vi "Process.vi"(8 "error in":errorcluster, 11 "Instrument":refnum<class "Instrument.lvclass">) -> (0 "error out":errorcluster, 3 "Instrument out":refnum<class "Instrument.lvclass">)   [LabVIEW 2019, in "Instrument.lvclass"]
doc: "---------------------------------------------------------------\nJKI State Machine Objects™\nhttp://jki.net/state-machine-objects/\nCopyright (C) 2005-2015, JKI <info@jki.net>\nALL RIGHTS RESERVED"
uses:
  Instrument.lvclass
  <vilib>/JKI/JKI SMO/SMO/SMO.lvclass
  <userlib>/LevyLab/RemoteControl/RemoteControl.lvclass
  <userlib>/LevyLab/RemoteControl/Typedefs/Message--Cluster.ctl
  <userlib>/LevyLab/RemoteControl/Typedefs/PrivateEvents--RemoteControl.Configure.ctl
  Logger.PGSQL/Logger.PGSQL.lvclass
  Logger.PGSQL/Typedefs/PrivateEvents--Logger.PGSQL.Write Variable.ctl
  C:/Program Files (x86)/National Instruments/LabVIEW 2019/vi.lib/JKI/JKI SMO/SMO/SMO.lvclass
  Logger.Error/Logger.Error.lvclass
panel:
  out "State History":string
  out "Local Command":string
  out "Name":string
  out "Remote Command":string
  # "1. Receives & processes commands from RemoteControl process\n2. Logs instrument settings to PGSQL using Logger process"
  # "INSTRUMENT"
  # "INSTRUMENT"
  # "For instructions on how to use the JKI State Machine Objects, examples and video tutorials, visit:\nhttp://jki.net/state-machine-objects/\n\nJKI State Machine Objects™\nhttp://jki.net/state-machine-objects/\nCopyright (C) 2005-2015, JKI <info@jki.net>\nALL RIGHTS RESERVED"
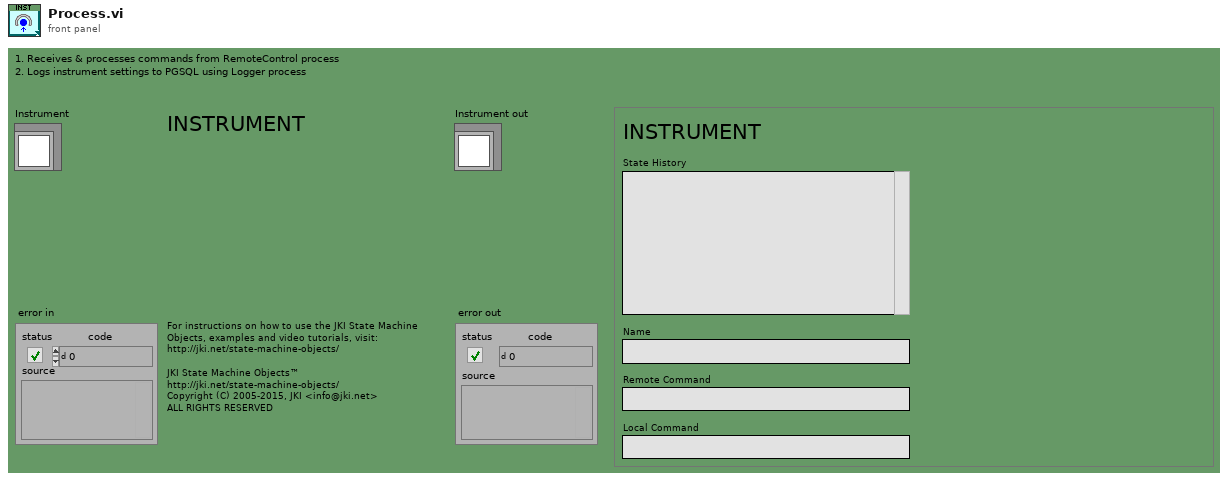
[diagram p1: front panel]
types:
  T1 = enum32{"invalid app kind", "Development System", "Run Time System", "Student Edition", "Embedded LabVIEW", "Evaluation", "Custom"}
  T2 = enum32{"Invalid", "Standard", "Closed", "Hidden", "Minimized", "Maximized"}
  T3 = typedef "RemoteControl.lvclass/Message--Cluster.ctl" = cluster{"Command":string, "Data":variant, "ID":string}
  T4 = typedef "Instrument.lvclass/Dependencies--Cluster.ctl" = cluster{"RemoteControl":refnum<class "RemoteControl.lvclass">, "Logger.Error":refnum<class "Logger.Error.lvclass">, "Logger.PGSQL":refnum<class "Logger.PGSQL.lvclass">, "Configuration":refnum<class "Configuration.lvclass">}
  T5 = typedef "RemoteControl.lvclass/PrivateEvents--RemoteControl.Configure.ctl" = cluster{"address":string, "Port":u16, "AllowedRemote":string, "Commands":string[], "timeout":i32}
  T6 = typedef "Logger.PGSQL.lvclass/PrivateEvents--Logger.PGSQL.Write Variable.ctl" = cluster{"Address":string, "Data":variant}
  T7 = cluster{"Core":cluster{"Current VI Reference":refnum<vi>, "Close Panel on Exit?":bool, "Last Error":cluster{"error":errorcluster, "previous state":string, "remaining states":string}, "Shutdown?":bool}, "SelfRef":refnum<class "Instrument.lvclass">, "Dependencies":T4, "RC Configuration":T5, "Message":T3, "getAll":variant, "Debug Mode?":bool, "PGSQL":T6}
  T8 = typedef "SMO.lvclass/SMOState --Enum.ctl" = enum16{"unknown", "Created", "Started", "Stopped"}
  T9 = cluster{"Current VI Reference":refnum<vi>, "Close Panel on Exit?":bool, "Last Error":cluster{"error":errorcluster, "previous state":string, "remaining states":string}, "Shutdown?":bool}
  T10 = typedef "SMO.lvclass/Protected Events.ctl" = cluster{"StopProcesses":refnum<user-event>, "AbortProcesses":refnum<user-event>, "Config Changed":refnum<user-event>, "Dependency":refnum<user-event>}
  T11 = typedef "Instrument.lvclass/PrivateEvents--Cluster.ctl" = cluster{"MessageToProcess":refnum<user-event>, "Log PGSQL":refnum<user-event>}
  T12 = typedef "RemoteControl.lvclass/PublicEvents--Cluster.ctl" = cluster{"SendMessageFromProcess":refnum<user-event>}
  T13 = typedef "SMO.lvclass/Public Events.ctl" = cluster{"Error":refnum<user-event>, "State":refnum<user-event>, "Reserve State":refnum<user-event>}
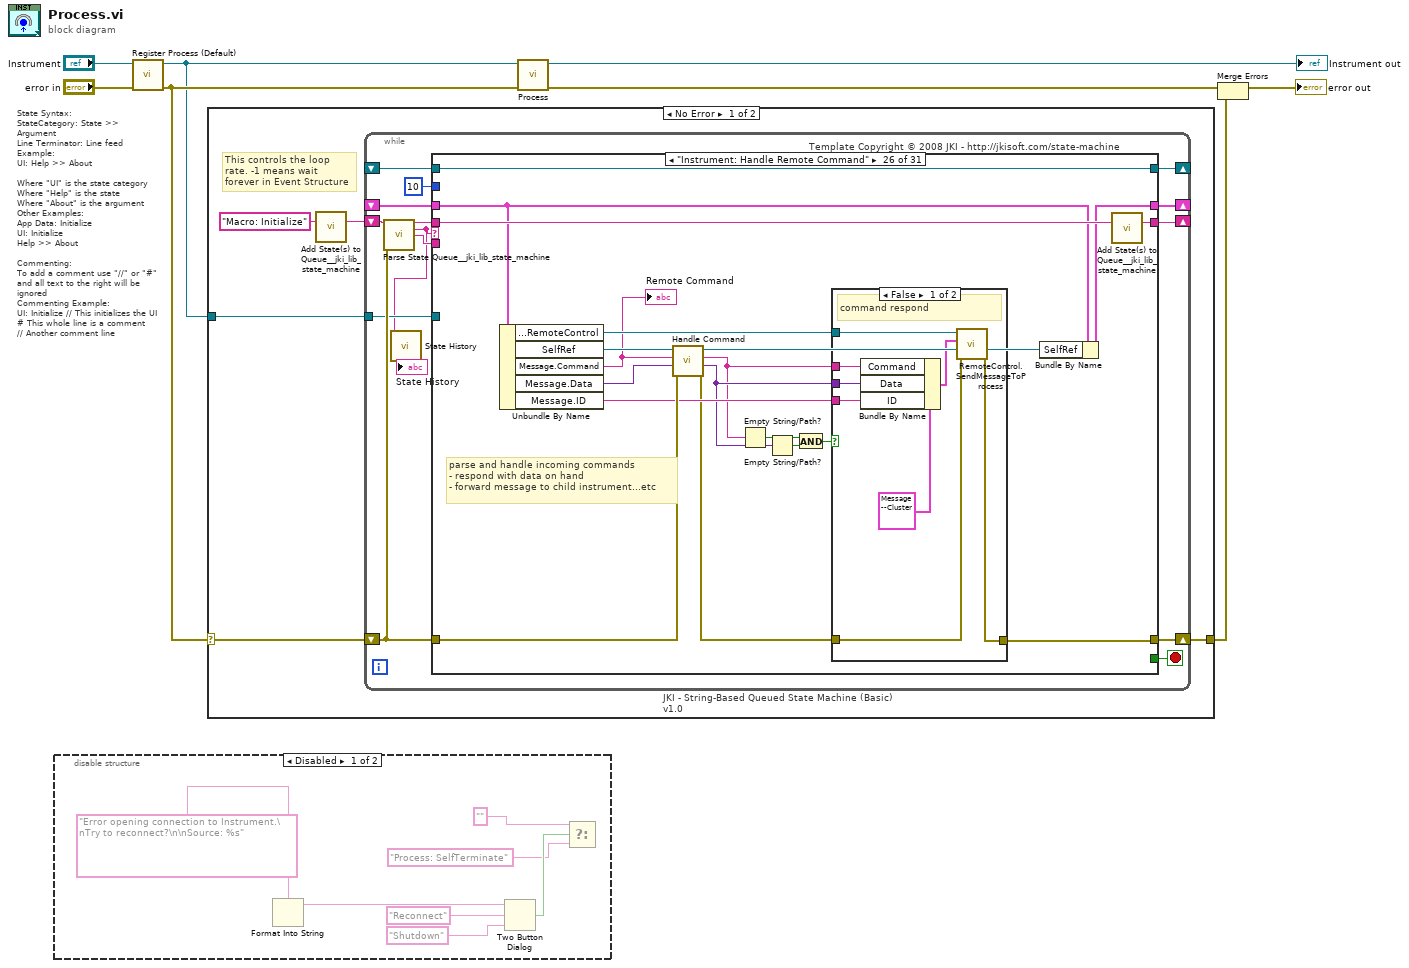
[diagram p0: block diagram]
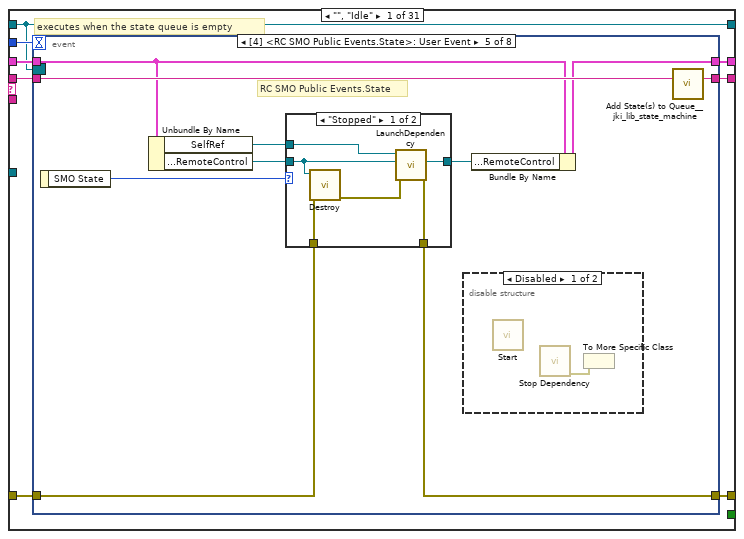
[diagram p3: hidden frame]
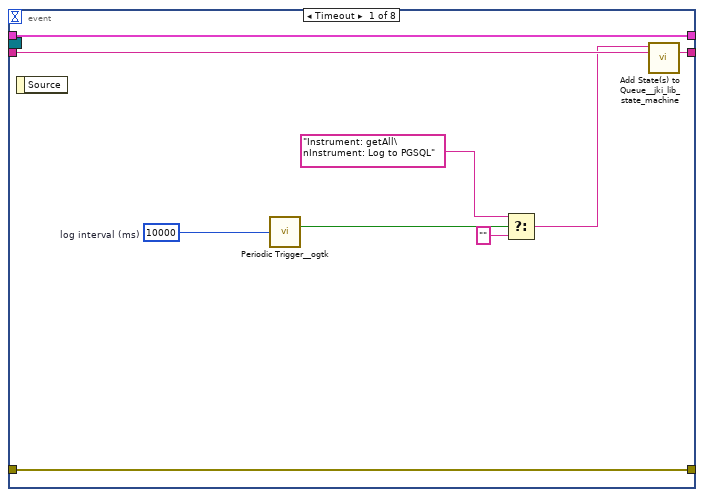
[diagram p4: hidden frame]
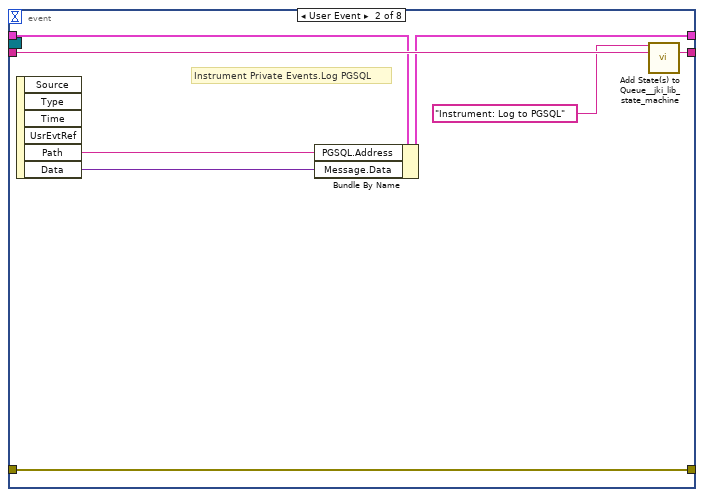
[diagram p5: hidden frame]
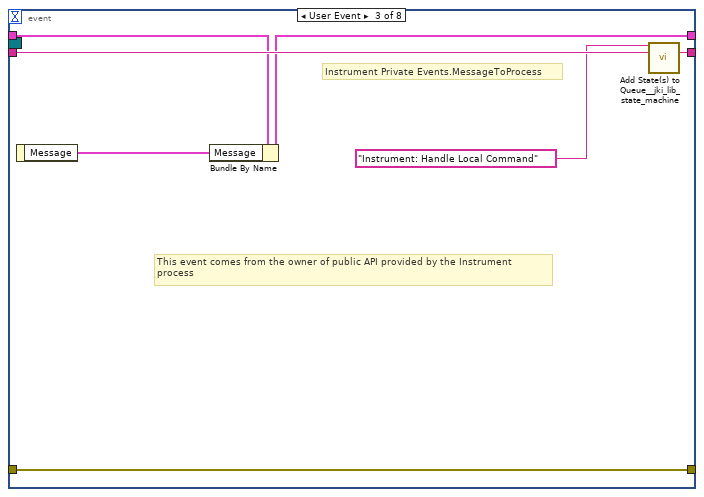
[diagram p6: hidden frame]
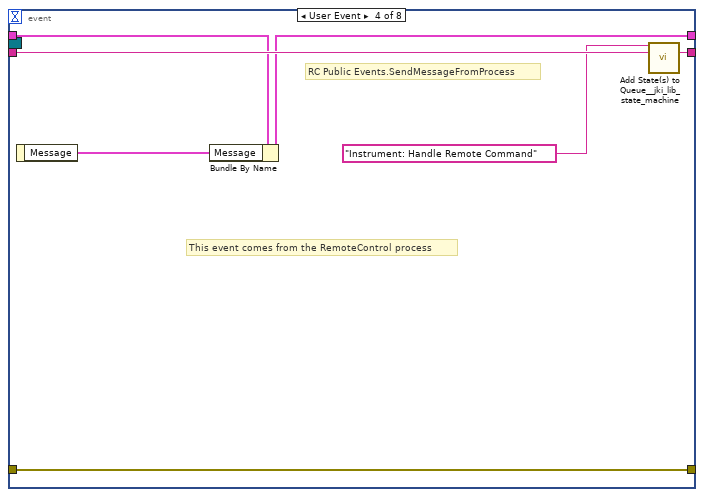
[diagram p7: hidden frame]
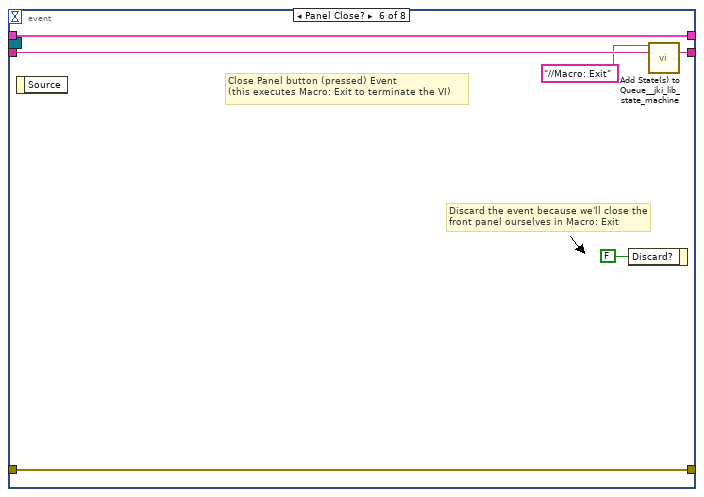
[diagram p10: hidden frame]
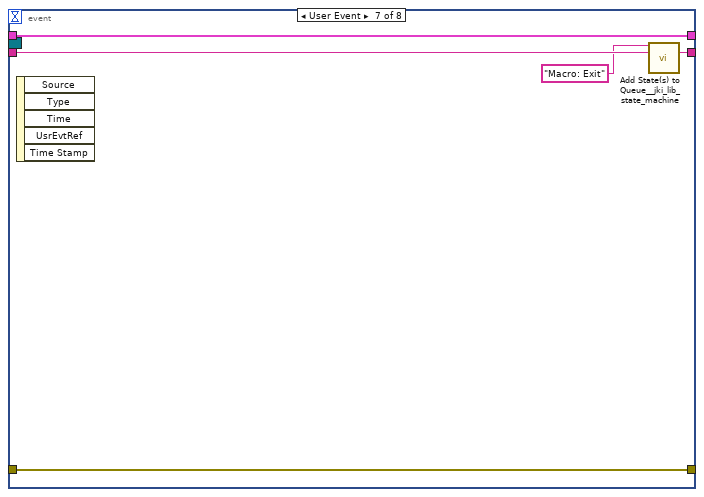
[diagram p11: hidden frame]
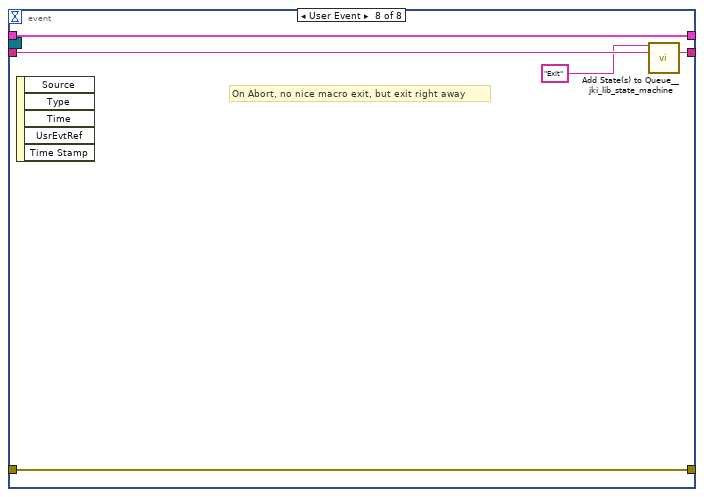
[diagram p12: hidden frame]
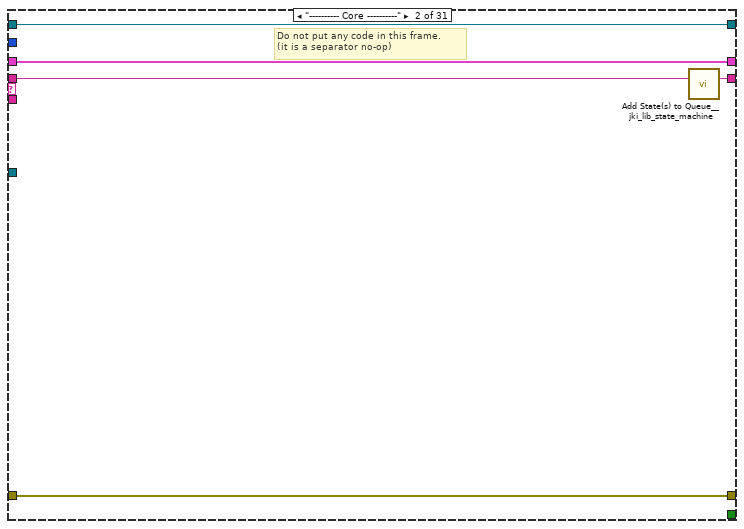
[diagram p13: hidden frame]
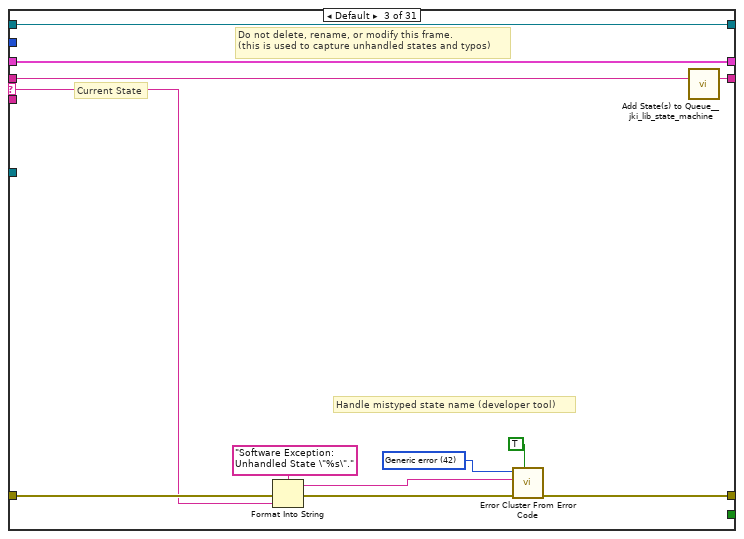
[diagram p14: hidden frame]
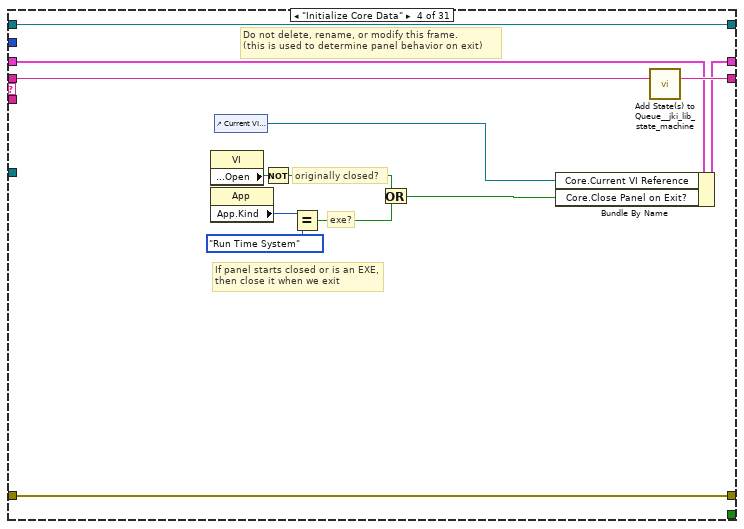
[diagram p15: hidden frame]
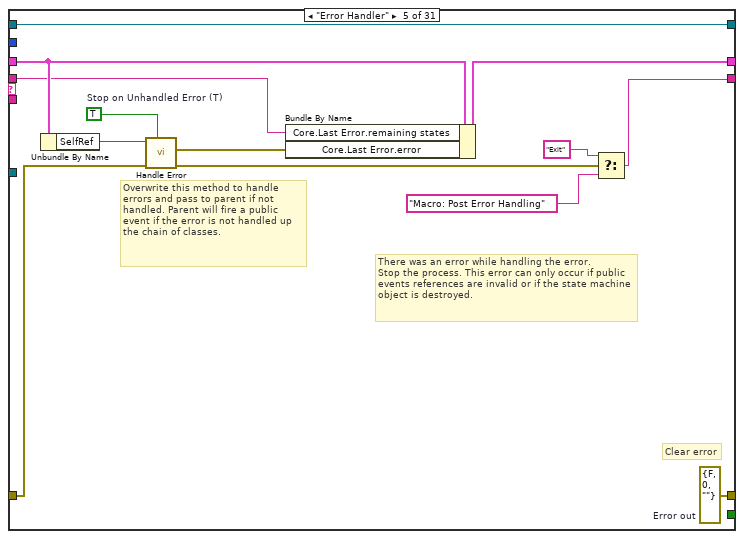
[diagram p16: hidden frame]
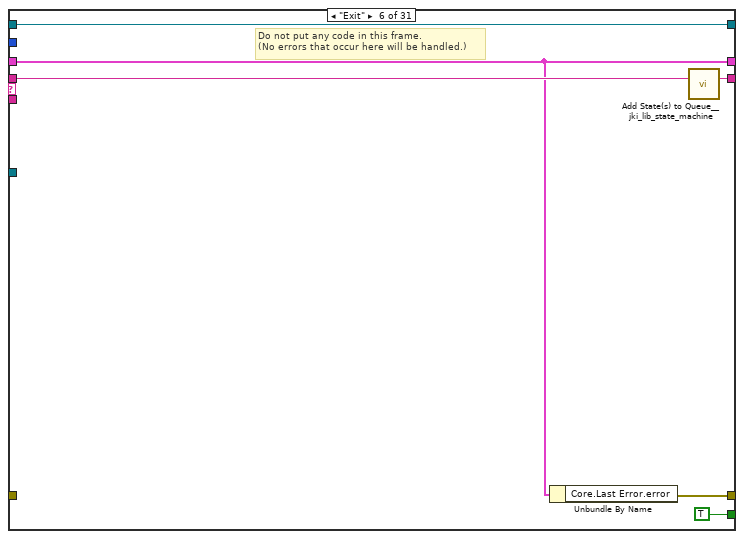
[diagram p17: hidden frame]
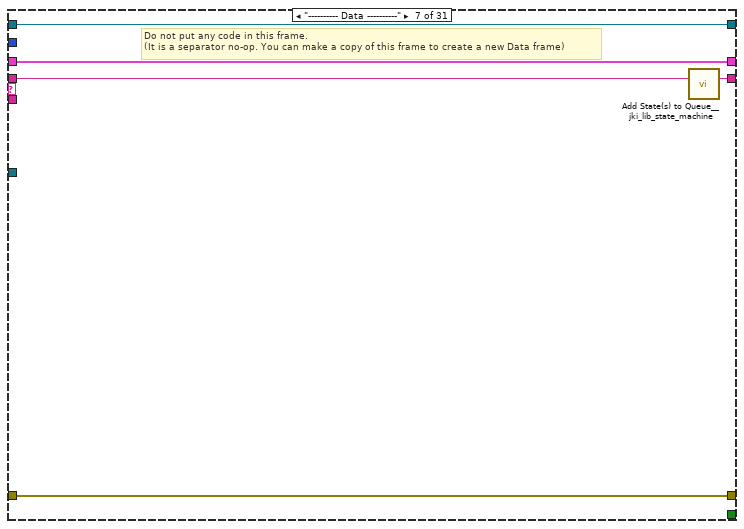
[diagram p18: hidden frame]
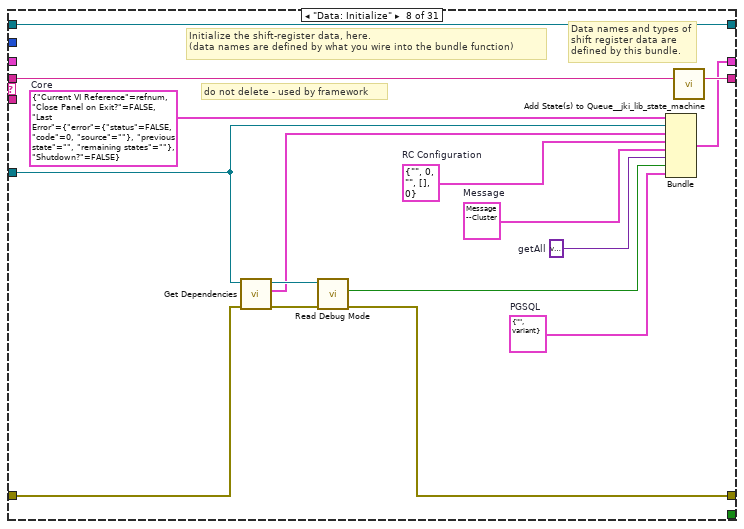
[diagram p19: hidden frame]
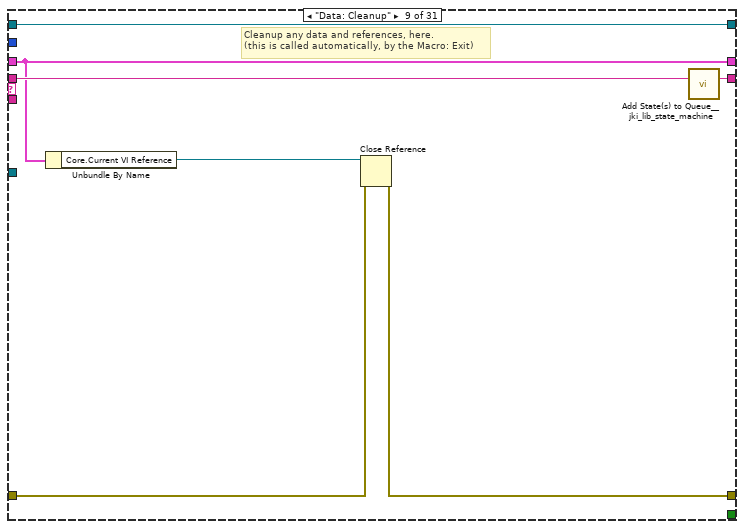
[diagram p20: hidden frame]
diagram:
  # "State Syntax:\nStateCategory: State >> Argument\nLine Terminator: Line feed\nExample:\nUI: Help >> About\n\nWhere \"UI\" is the state category\nWhere \"Help\" is the state\nWhere \"About\" is the argument\nOther Examples:\nApp Data: Initialize\nUI: Initialize\nHelp >> About\n\nCommenting:\nTo add a comment use \"//\" or \"#\" and all text to the right will be ignored\nCommenting Example:\nUI: Initialize // This initializes the UI\n# This whole line is a comment\n// Another comment line"
  n1 = disable-structure shown="Disabled" {
    frame Disabled {
      n2 = Format Into String(format string="Error opening connection to Instrument.\nTry to reconnect?\n\nSource: %s" ("message")) -> (resulting string=w9:string)  [unwired: 3 in, 1 out]
      n3 = Two Button Dialog(message=w9, 1:"Shutdown" ("F button name (\"Cancel\")"), 2:"Reconnect" ("T button name (\"OK\")")) -> (T button?=w13:bool)
      n4 = Select(t="" ("States to Execute"), s=w13, f="Process: SelfTerminate" ("States to Execute")) -> ()  [unwired: 1 out]
    }
    frame Enabled {
    }
  }
  n5 = call <vilib>:"Register Process (Default).vi"("error in (no error)"="error in", "SMO"="Instrument") -> ("error out"=w5:errorcluster, "SelfRef"=w4:refnum<class "Instrument.lvclass">)  [unwired: 8 in]
  n6 = case shown="No Error" w5 {
    selector: w5 -> [w17 w513]
    tunnel: w4 -> [w18 _]
    tunnel: [w16 w513] -> w1
    frame No Error {
      # "This controls the loop rate. -1 means wait forever in Event Structure"
      n7 = call <vilib>:"Add State(s) to Queue__jki_lib_state_machine.vi"("State(s) in (\"\")"="Macro: Initialize") -> ("States Out"=w20:string)  [unwired: 14 in]
      n8 = while "JKI - String-Based Queued State Machine (Basic) v1.0" {
        shift-right: [w29] -> _
        shift-left: _ -> [w28]
        shift-right: [w32] -> w16
        shift-left: w17 -> [w26]
        shift-right: [w31] -> _
        shift-left: w20 -> [w33]
        tunnel: w18 -> [w23]
        shift-right: [w25] -> _
        shift-left: _ -> [w24]
        stop <- w30 stop-if-true
        # "Template Copyright © 2008 JKI - http://jkisoft.com/state-machine"
        n9 = call <vilib>:"Parse State Queue__jki_lib_state_machine.vi"("State Queue"=w33, "Error In (no error)"=w26) -> ("Remaining States"=w35:string, "Current State"=w22:string, "Arguments"=w34:string)  [unwired: 11 in]
        n10 = call "State History.vi"("Current State"=w22) -> ("History"=→"State History":string)  [unwired: 10 in]
        n11 = case shown="\"Instrument: Handle Remote Command\"" w22 {
          selector: w22 -> [_ _ w116 _ _ _ _ _ _ _ _ _ _ _ _ _ _ _ _ _ _ _ _ _ _ _ _ _ _ _ _]
          tunnel: w35 -> [w43 w114 w120 w139 w141 w158 w163 w179 w186 w191 w201 w208 w224 w261 w266 w283 w302 w306 w323 w334 w343 w348 w379 w385 w390 w409 w437 w461 w482 w491 w506]
          tunnel: w34 -> [_ _ _ _ _ _ _ _ _ _ _ w202 w218 _ _ _ _ _ _ _ _ _ _ _ _ _ _ _ _ _ _]
          tunnel: w28 -> [w41 w111 w118 w130 w150 w154 w160 _ w181 w188 w198 w206 w220 w256 w263 w277 w294 w309 w320 w331 w338 w345 w377 w383 w388 w401 w426 w451 w476 w487 w500]
          tunnel: [w40 w112 w122 w136 w151 w153 w161 w169 w182 w189 w192 w203 w221 w257 w264 w274 w300 w313 w321 w325 w335 w346 w375 w381 w386 w392 w431 w455 w477 w484 w499] -> w32
          tunnel: w26 -> [w39 w112 w121 w136 w142 _ w161 w164 w183 w189 w195 w204 w222 w258 w264 w275 w300 w313 w321 w326 w336 w346 w373 w381 w386 w405 w434 w458 w478 w483 w498]
          tunnel: [w42 w113 w119 w138 w146 w157 w162 w178 w185 w190 w200 w207 w223 w260 w265 w282 w301 w307 w322 w333 w342 w347 w378 w384 w389 w408 w436 w460 w481 w490 w505] -> w31
          tunnel: [_ _ _ _ _ TRUE _ _ _ _ _ _ _ _ _ _ _ _ _ _ _ _ _ _ _ _ _ _ _ _ _] -> w30
          tunnel: [w38 w111 w118 w137 w149 w154 w160 w177 w181 w188 w198 w206 w220 w256 w263 w277 w294 w310 w320 w331 w337 w345 w377 w383 w388 w400 w425 w450 w476 w488 w501] -> w29
          tunnel: 10 ("Timeout") -> [w37 _ _ _ _ _ _ _ _ _ _ _ _ _ _ _ _ _ _ _ _ _ _ _ _ _ _ _ _ _ _]
          tunnel: [w36 w110 w115 w127 w152 w155 w159 w176 w180 w187 w199 w205 w217 w259 w262 w281 w295 w314 w319 w332 w341 w344 w376 w382 w387 w407 w435 w459 w480 w489 w504] -> w25
          tunnel: w24 -> [w36 w110 w115 w127 w152 w155 w159 w176 w180 w187 w199 w205 w217 w259 w262 w281 w295 w314 w319 w332 w341 w344 _ w382 w387 w407 w435 w459 w480 w489 w504]
          tunnel: w23 -> [_ _ _ _ _ _ _ w165 _ _ _ _ _ _ _ w276 _ _ _ _ _ _ _ _ _ _ _ _ _ _ _]
          frame "", "Idle" {
            # "executes when the state queue is empty"
            n12 = event shown="[4] <RC SMO Public Events.State>: User Event" {
              selector: w36 -> [_ _ _ _ _ _ _ _]
              dyn-events: _ -> [_ _ _ _ _ _ _ _]
              timeout: w37 -> [_ _ _ _ _ _ _ _]
              tunnel: w43 -> [w52 w60 w67 w74 w84 w99 w104 w109]
              tunnel: [w51 w59 w66 w73 w83 w98 w103 w108] -> w42
              tunnel: w41 -> [w45 w55 w64 w71 w79 w96 w101 w106]
              tunnel: [w50 w58 w65 w72 w76 w97 w102 w107] -> w40
              tunnel: w39 -> [w50 w58 w65 w72 w77 w97 w102 w107]
              tunnel: [w45 w54 w63 w70 w78 w96 w101 w106] -> w38
              event Timeout {
                w46 = u32 10000  # log interval (ms)
                n13 = event-data() -> ()  [unwired: 1 in, 1 out]
                n14 = call <userlib>:"Periodic Trigger__ogtk.vi"("time (ms)"=w46) -> ("Triggered"=w48:bool)  [unwired: 12 in, 2 out]
                n15 = Select(t="Instrument: getAll\nInstrument: Log to PGSQL" ("State(s) in Front (\"\")"), s=w48, f="") -> (s? t:f=w49:string)
                n16 = call <vilib>:"Add State(s) to Queue__jki_lib_state_machine.vi"("State(s) in Front (\"\")"=w49, "State(s) in (\"\")"=w52) -> ("States Out"=w51:string)  [unwired: 13 in]
              }
              event User Event {
                # "Instrument Private Events.Log PGSQL"
                n17 = event-data() -> ("Path"=w57:string, "Data"=w56:variant)  [unwired: 1 in, 4 out]
                n18 = Bundle By Name(cluster=w55, "PGSQL.Address"=w57, "Message.Data"=w56) -> (w54:T7)
                n19 = call <vilib>:"Add State(s) to Queue__jki_lib_state_machine.vi"("State(s) in Front (\"\")"="Instrument: Log to PGSQL" ("State(s) in Front (\"\")"), "State(s) in (\"\")"=w60) -> ("States Out"=w59:string)  [unwired: 13 in]
              }
              event User Event {
                # "Instrument Private Events.MessageToProcess"
                # "This event comes from the owner of public API provided by the Instrument\nprocess"
                n20 = event-data() -> ("Message"=w62:T3)  [unwired: 1 in]
                n21 = Bundle By Name(cluster=w64, "Message"=w62) -> (w63:T7)
                n22 = call <vilib>:"Add State(s) to Queue__jki_lib_state_machine.vi"("State(s) in Front (\"\")"="Instrument: Handle Local Command" ("State(s) in Front (\"\")"), "State(s) in (\"\")"=w67) -> ("States Out"=w66:string)  [unwired: 13 in]
              }
              event User Event {
                # "RC Public Events.SendMessageFromProcess"
                # "This event comes from the RemoteControl process"
                n23 = event-data() -> ("Message"=w69:T3)  [unwired: 1 in]
                n24 = Bundle By Name(cluster=w71, "Message"=w69) -> (w70:T7)
                n25 = call <vilib>:"Add State(s) to Queue__jki_lib_state_machine.vi"("State(s) in Front (\"\")"="Instrument: Handle Remote Command" ("State(s) in Front (\"\")"), "State(s) in (\"\")"=w74) -> ("States Out"=w73:string)  [unwired: 13 in]
              }
              event User Event {
                # "RC SMO Public Events.State"
                n26 = event-data() -> ("SMO State"=w82:T8)  [unwired: 1 in]
                n27 = Unbundle By Name(w79) -> ("SelfRef"=w75:refnum<class "Instrument.lvclass">, "Dependencies.RemoteControl"=w81:refnum<class "RemoteControl.lvclass">)
                n28 = case shown="\"Stopped\"" w82 {
                  tunnel: w81 -> [w86 w93]
                  tunnel: [w91 w93] -> w80
                  tunnel: w77 -> [w88 w92]
                  tunnel: [w90 w92] -> w76
                  tunnel: w75 -> [w89 _]
                  frame "Stopped" {
                    n29 = call <vilib>:"Destroy.vi"("error in (no error)"=w88, "SMO"=w86) -> ("error out"=w87:errorcluster)  [unwired: 9 in]
                    n30 = call <vilib>:"LaunchDependency.vi"("error in (no error)"=w87, "Dependency Type"=w86, "SMO in"=w89) -> ("error out"=w90:errorcluster, "Dependency Reference"=w91:refnum<class "RemoteControl.lvclass">)  [unwired: 5 in, 2 out]
                  }
                  frame Default {
                  }
                }
                n31 = disable-structure shown="Disabled" {
                  frame Disabled {
                    n32 = call <vilib>:"Start.vi"() -> ()  [unwired: 10 in, 2 out]
                    n33 = call <vilib>:"Stop Dependency.vi"() -> ("error out"=w85:errorcluster)  [unwired: 9 in, 2 out]
                    n34 = To More Specific Class(error in=w85) -> ()  [unwired: 2 in, 2 out]
                  }
                  frame Enabled {
                  }
                }
                n35 = Bundle By Name(cluster=w79, "Dependencies.RemoteControl"=w80) -> (w78:T7)
                n36 = call <vilib>:"Add State(s) to Queue__jki_lib_state_machine.vi"("State(s) in (\"\")"=w84) -> ("States Out"=w83:string)  [unwired: 14 in]
              }
              event Panel Close? {
                # "Discard the event because we'll close the front panel ourselves in Macro: Exit"
                # "Close Panel button (pressed) Event\n(this executes Macro: Exit to terminate the VI)"
                n37 = event-data() -> ()  [unwired: 1 in, 1 out]
                n38 = event-data("Discard?"=FALSE) -> ()  [unwired: 1 in, 1 out]
                n39 = call <vilib>:"Add State(s) to Queue__jki_lib_state_machine.vi"("State(s) in Front (\"\")"="//Macro: Exit", "State(s) in (\"\")"=w99) -> ("States Out"=w98:string)  [unwired: 13 in]
              }
              event User Event {
                n40 = event-data() -> ()  [unwired: 1 in, 5 out]
                n41 = call <vilib>:"Add State(s) to Queue__jki_lib_state_machine.vi"("State(s) in Front (\"\")"="Macro: Exit", "State(s) in (\"\")"=w104) -> ("States Out"=w103:string)  [unwired: 13 in]
              }
              event User Event {
                # "On Abort, no nice macro exit, but exit right away"
                n42 = event-data() -> ()  [unwired: 1 in, 5 out]
                n43 = call <vilib>:"Add State(s) to Queue__jki_lib_state_machine.vi"("State(s) in Front (\"\")"="Exit", "State(s) in (\"\")"=w109) -> ("States Out"=w108:string)  [unwired: 13 in]
              }
            }
          }
          frame "---------- Core ----------" {
            # "Do not put any code in this frame.\n(it is a separator no-op)"
            n44 = call <vilib>:"Add State(s) to Queue__jki_lib_state_machine.vi"("State(s) in (\"\")"=w114) -> ("States Out"=w113:string)  [unwired: 14 in]
          }
          frame Default {
            w125 = 42 items=["No error", "Argument error", "Memory is full", "Out of zone", "End of file", "File already open", "Generic file I/O error", "File not found", "File permission error", "Disk is full", "Duplicate path", "Too many files open", "System feature not enabled", "Resource file not found", "Cannot add resource", "Resource not found", "Image not found", "Image memory error", "Pen does not exist", "Config type invalid", "Config token not found", "Config parse error", "Config memory error", "Bad external code format", "Bad external code offset", "External code not present", "Null window", "Destroy window error", "Null menu", "Print aborted", "Bad print record", "Print driver error", "Windows error during printing", "Memory error during printing", "Print dialog error", "Generic print error", "Invalid device refnum", "Device not found", "Device parameter error", "Device unit error", "Cannot open device", "Device call aborted", "Generic error", "Cancelled by user", "Object ID too low", "Object ID too high", "Object not in heap", "Unknown heap", "Unknown object (invalid DefProc)", "Unknown object (DefProc not in table)", "Message out of range", "Invalid (null) method", "Unknown message", "Manager call not supported", "Bad address", "Network operation in progress", "Network operation timed out", "Connection is busy", "Network attribute not supported", "Network error", "Address in use", "System out of memory", "Connection aborted", "Connection refused", "Not connected", "Already connected", "Connection closed", "Initialization error (interapplication manager)", "Bad occurrence", "Wait on unbound occurrence handler", "Occurrence queue overflow", "Datalog type conflict", "Unused", "Unrecognized type (interapplication manager)", "Memory corrupt", "Failed to make temporary DLL", "Old CIN version", "Drag socket not found", "Failed to load drop-object", "Failed to register OLE object", "Failed to release OLE object", "Format specifier type mismatch", "Unknown format specifier", "Too few format specifiers", "Too many format specifiers", "Scan failed", "Newer CIN version", "Error converting to variant", "Runtime menu error", "Password tampered", "Variant attribute not found", "Incompatible variant data type", "Event data is not available", "Event Store is not present", "Occurrence is not found", "Event Queue is not created", "Event info is not available", "Refnum passed is NULL", "Error retrieving Class GUID", "Error retrieving CoClass GUID", "Error retrieving TypeLib GUID.", "Bad built application magic bytes.", "Specific driver is different from the specific driver associated with the Logical Name.", "There is no session opened to the class driver.", "Max Error", "MAX - Error with config objects", "MAX - Error loading configuration", "MAX - Group not supported"]
            # "Current State"
            # "Do not delete, rename, or modify this frame.\n(this is used to capture unhandled states and typos)"
            # "Handle mistyped state name (developer tool)"
            n45 = Format Into String(format string="Software Exception: Unhandled State \"%s\"." ("message"), error in=w121, w116) -> (resulting string=w124:string, error out=w123:errorcluster)  [unwired: 1 in]
            n46 = call <vilib>:"Error Cluster From Error Code.vi"("show call chain? (False)"=TRUE, "error in (no error)"=w123, "error message (\"\")"=w124, "error code (0)"=w125) -> ("error out"=w122:errorcluster)  [unwired: 5 in]
            n47 = call <vilib>:"Add State(s) to Queue__jki_lib_state_machine.vi"("State(s) in (\"\")"=w120) -> ("States Out"=w119:string)  [unwired: 14 in]
          }
          frame "Initialize Core Data" {
            # "Do not delete, rename, or modify this frame.\n(this is used to determine panel behavior on exit)"
            # "originally closed?"
            # "exe?"
            # "If panel starts closed or is an EXE, then close it when we exit"
            n48 = property class="VI"() -> ("Front Panel.Open"=w135:bool)  [unwired: 2 in, 2 out]
            n49 = property class="App"() -> ("App.Kind"=w134:T1)  [unwired: 2 in, 2 out]
            n50 = control-ref of="Current VI Reference"() -> (w128:refnum<vi>)
            n51 = Not(x=w135) -> (.not. x?=w132:bool)
            n52 = Equal?(x=w134, y=T1."Run Time System" ("Application:Kind")) -> (x = y?=w131:bool)
            n53 = Or(x=w132, y=w131) -> (x .or. y?=w129:bool)
            n54 = Bundle By Name(cluster=w130, "Core.Current VI Reference"=w128, "Core.Close Panel on Exit?"=w129) -> (w137:T7)
            n55 = call <vilib>:"Add State(s) to Queue__jki_lib_state_machine.vi"("State(s) in (\"\")"=w139) -> ("States Out"=w138:string)  [unwired: 14 in]
          }
          frame "Error Handler" {
            w147 = TRUE  # Stop on Unhandled Error (T)
            w151 = errorcluster {"status"=FALSE, "code"=0, "source"=""}  # Error out
            # "Clear error"
            # "There was an error while handling the error.\nStop the process. This error can only occur if public events references are invalid or if the state machine object is destroyed."
            # "Overwrite this method to handle errors and pass to parent if not handled. Parent will fire a public event if the error is not handled up the chain of classes."
            n56 = Unbundle By Name(w150) -> ("SelfRef"=w143:refnum<class "Instrument.lvclass">)
            n57 = call-dynamic "Handle Error.vi"("Stop on Unhandled Error (T)"=w147, "error in"=w142, "SMO"=w143) -> ("handling error"=w144:errorcluster, "Unhandled error"=w145:errorcluster)  [unwired: 6 in, 1 out]
            n58 = Bundle By Name(cluster=w150, "Core.Last Error.remaining states"=w141, "Core.Last Error.error"=w145) -> (w149:T7)
            n59 = Select(t="Exit", s=w144, f="Macro: Post Error Handling" ("State")) -> (s? t:f=w146:string)
          }
          frame "Exit" {
            # "Do not put any code in this frame.\n(No errors that occur here will be handled.)"
            n60 = Unbundle By Name(w154) -> ("Core.Last Error.error"=w153:errorcluster)
            n61 = call <vilib>:"Add State(s) to Queue__jki_lib_state_machine.vi"("State(s) in (\"\")"=w158) -> ("States Out"=w157:string)  [unwired: 14 in]
          }
          frame "---------- Data ----------" {
            # "Do not put any code in this frame.\n(It is a separator no-op. You can make a copy of this frame to create a new Data frame)"
            n62 = call <vilib>:"Add State(s) to Queue__jki_lib_state_machine.vi"("State(s) in (\"\")"=w163) -> ("States Out"=w162:string)  [unwired: 14 in]
          }
          frame "Data: Initialize" {
            w167 = T6 {"Address"="", "Data"=variant}  # PGSQL
            w172 = variant  # getAll
            w173 = T5 {"address"="", "Port"=0, "AllowedRemote"="", "Commands"=[], "timeout"=0}  # RC Configuration
            w174 = T3 {"Command"="", "Data"=variant(string ""), "ID"=""}  # Message
            w175 = T9 {"Current VI Reference"=refnum, "Close Panel on Exit?"=FALSE, "Last Error"={"error"={"status"=FALSE, "code"=0, "source"=""}, "previous state"="", "remaining states"=""}, "Shutdown?"=FALSE}  # Core
            # "do not delete - used by framework"
            # "Data names and types of shift register data are defined by this bundle."
            # "Initialize the shift-register data, here.\n(data names are defined by what you wire into the bundle function)"
            n63 = call "Get Dependencies.vi"("error in (no error)"=w164, "Instrument in"=w165) -> ("error out"=w170:errorcluster, "Dependencies"=w166:T4, "Instrument out"=w171:refnum<class "Instrument.lvclass">)  [unwired: 7 in]
            n64 = call-dynamic "Read Debug Mode.vi"("error in (no error)"=w170, "Instrument in"=w171) -> ("error out"=w169:errorcluster, "Debug Mode?"=w168:bool)  [unwired: 7 in, 1 out]
            n65 = Bundle("Core"=w175, "SelfRef"=w165, "Dependencies"=w166, "RC Configuration"=w173, "Message"=w174, "getAll"=w172, "Debug Mode?"=w168, "PGSQL"=w167) -> (w177:T7)  [unwired: 1 in]
            n66 = call <vilib>:"Add State(s) to Queue__jki_lib_state_machine.vi"("State(s) in (\"\")"=w179) -> ("States Out"=w178:string)  [unwired: 14 in]
          }
          frame "Data: Cleanup" {
            # "Cleanup any data and references, here.\n(this is called automatically, by the Macro: Exit)"
            n67 = Unbundle By Name(w181) -> ("Core.Current VI Reference"=w184:refnum<vi>)
            n68 = Close Reference(reference=w184, error in (no error)=w183) -> (error out=w182:errorcluster)
            n69 = call <vilib>:"Add State(s) to Queue__jki_lib_state_machine.vi"("State(s) in (\"\")"=w186) -> ("States Out"=w185:string)  [unwired: 14 in]
          }
          frame "---------- UI ----------" {
            # "Do not put any code in this frame.\n(It is a separator no-op. You can make a copy of this frame to create a new UI frame)"
            n70 = call <vilib>:"Add State(s) to Queue__jki_lib_state_machine.vi"("State(s) in (\"\")"=w191) -> ("States Out"=w190:string)  [unwired: 14 in]
          }
          frame "UI: Initialize" {
            # "Initialize the User Interface, here.\n(this is called automatically, by the Macro: Init)"
            n71 = Unbundle By Name(w198) -> ("SelfRef"=w197:refnum<class "Instrument.lvclass">)
            n72 = call <vilib>:"GetName.vi"("error in (no error)"=w195, "SMO"=w197) -> ("error out"=w193:errorcluster, "Name"=→"Name":string)  [unwired: 6 in, 2 out]
            n73 = call <userlib>:"Fit VI window to Largest Dec__ogtk.vi"("error in (no error)"=w193, "border spacing (2 px)"=0) -> ("error out"=w192:errorcluster)  [unwired: 4 in, 1 out]
            n74 = call <vilib>:"Add State(s) to Queue__jki_lib_state_machine.vi"("State(s) in (\"\")"=w201) -> ("States Out"=w200:string)  [unwired: 14 in]
          }
          frame "UI: Cursor Set" {
            # "Argument"
            # "Initialize the User Interface, here.\n(this is called automatically, by the Macro: Init)"
            n75 = disable-structure shown="Default" {
              disable-tunnel: w204 -> [w209 w212]
              disable-tunnel: [w209 w211] -> w203
              disable-tunnel: w202 -> [_ w210]
              frame condition #0 {
              }
              frame condition #1 (active) {
                n76 = case shown="\"Busy\"" w210 {
                  tunnel: w212 -> [w214 w216]
                  tunnel: [w213 w215] -> w211
                  frame "Idle", Default {
                    n77 = call <vilib>:"Unset Busy.vi"("error in (no error)"=w214) -> ("error out"=w213:errorcluster)  [unwired: 10 in]
                  }
                  frame "Busy" {
                    n78 = call <vilib>:"Set Busy.vi"("error in (no error)"=w216) -> ("error out"=w215:errorcluster)  [unwired: 9 in, 1 out]
                  }
                }
              }
            }
            n79 = call <vilib>:"Add State(s) to Queue__jki_lib_state_machine.vi"("State(s) in (\"\")"=w208) -> ("States Out"=w207:string)  [unwired: 14 in]
          }
          frame "UI: Front Panel State" {
            # "Argument"
            # "Set Front Panel Open or Closed\n(Usage: \"UI: Front Panel State >> Open|Close\")"
            n80 = Unbundle By Name(w220) -> ("Core.Current VI Reference"=w219:refnum<vi>)
            n81 = disable-structure shown="Default" {
              disable-tunnel: w222 -> [w228 w251]
              disable-tunnel: [w227 w251] -> w221
              disable-tunnel: w219 -> [w226 _]
              disable-tunnel: w218 -> [w225 _]
              frame condition #0 (active) {
                n82 = case shown="\"Close\"" w225 {
                  tunnel: w228 -> [w232 w245]
                  tunnel: [w234 w246] -> w227
                  tunnel: w226 -> [w233 w243]
                  frame "Open", Default {
                    n83 = property class="VI"(reference=w233, error in=w232) -> (reference out=w230:refnum<vi>, error out=w231:errorcluster, "FP.State"=w229:T2)
                    n84 = case shown="Default" w229 {
                      tunnel: [w237 w240] -> w234
                      tunnel: w231 -> [w236 w240]
                      tunnel: w230 -> [w235 _]
                      frame "Closed" {
                        n85 = invoke class="VI" method="FP.Open"(reference=w235, error in=w236, "Activate"=TRUE, "State"=T2."Standard") -> (error out=w237:errorcluster)  [unwired: 1 in, 4 out]
                      }
                      frame Default {
                      }
                    }
                  }
                  frame "Close" {
                    n86 = property class="VI"(reference=w243, error in=w245) -> (reference out=w242:refnum<vi>, error out=w244:errorcluster, "FP.State"=w241:T2)
                    n87 = case shown="Default" w241 {
                      tunnel: [w247 w250] -> w246
                      tunnel: w244 -> [w247 w249]
                      tunnel: w242 -> [_ w248]
                      frame "Invalid", "Closed" {
                      }
                      frame Default {
                        n88 = invoke class="VI" method="FP.Close"(reference=w248, error in=w249) -> (error out=w250:errorcluster)  [unwired: 1 in, 2 out]
                      }
                    }
                  }
                }
              }
              frame condition #1 {
              }
            }
            n89 = call <vilib>:"Add State(s) to Queue__jki_lib_state_machine.vi"("State(s) in (\"\")"=w224) -> ("States Out"=w223:string)  [unwired: 14 in]
          }
          frame "UI: Wait" {
            n90 = Unbundle By Name(w256) -> ("Debug Mode?"=w253:bool)
            n91 = Select(t=u32 5000 ("milliseconds to wait"), s=w253, f=u32 0 ("milliseconds to wait")) -> (s? t:f=w252:u32)
            n92 = call <userlib>:"Wait (ms)__ogtk.vi"("error in (no error)"=w258, "milliseconds to wait"=w252) -> ("error out"=w257:errorcluster)  [unwired: 8 in, 1 out]
            n93 = call <vilib>:"Add State(s) to Queue__jki_lib_state_machine.vi"("State(s) in (\"\")"=w261) -> ("States Out"=w260:string)  [unwired: 14 in]
          }
          frame "---------- Macro ----------" {
            # "Do not put any code in this frame.\n(It is a separator no-op. You can make a copy of this frame to create a new Macro frame)"
            n94 = call <vilib>:"Add State(s) to Queue__jki_lib_state_machine.vi"("State(s) in (\"\")"=w266) -> ("States Out"=w265:string)  [unwired: 14 in]
          }
          frame "Macro: Initialize" {
            # "This needs to be called here before Data: Initialize\nto ensure that the correct argument"
            # "Initialization Macro\n(This is called once, when the VI starts)"
            n95 = call-dynamic "Read Debug Mode.vi"("error in (no error)"=w275, "Instrument in"=w276) -> ("error out"=w274:errorcluster, "Debug Mode?"=w273:bool)  [unwired: 7 in, 1 out]
            n96 = Select(t="Open", s=w273, f="Close") -> (s? t:f=w270:string)
            n97 = Format Into String(format string="UI: Initialize\nUI: Front Panel State >> %s\nUI: Wait\nInstrument: Open", initial string="", w270) -> (resulting string=w269:string)  [unwired: 1 in, 1 out]
            n98 = call <vilib>:"Add State(s) to Queue__jki_lib_state_machine.vi"("State(s) in Front (\"\")"="Data: Initialize\nInitialize Core Data\nEvents: Register", "State(s) in (\"\")"="Process: Sync", "State(s) at Back (\"\")"=w269) -> ("States Out"=w279:string)  [unwired: 12 in]
            n99 = call <vilib>:"Add State(s) to Queue__jki_lib_state_machine.vi"("State(s) in Front (\"\")"=w279, "State(s) in (\"\")"=w283) -> ("States Out"=w282:string)  [unwired: 13 in]
          }
          frame "Macro: Exit" {
            # "Exit Macro\n(This is called once, when the VI exits)"
            n100 = Unbundle By Name(w294) -> ("Debug Mode?"=w288:bool, "Core.Close Panel on Exit?"=w299:bool)
            n101 = Select(t="Open", s=w288, f="Close") -> (s? t:f=w285:string)
            n102 = call <vilib>:"Build State String with Arguments__JKI_lib_State_Machine.vi"("Arguments (\"\")"=w285, "State"="UI: Front Panel State") -> ("State with Arguments"=w289:string)  [unwired: 4 in]
            n103 = Select(t=w289, s=w299, f="") -> (s? t:f=w297:string)
            n104 = call <vilib>:"Add State(s) to Queue__jki_lib_state_machine.vi"("State(s) in Front (\"\")"="Instrument: Close\nData: Cleanup\nEvents: Unregister", "State(s) in (\"\")"="Process: Sync", "State(s) at Back (\"\")"="Exit") -> ("States Out"=w291:string)  [unwired: 12 in]
            n105 = call <vilib>:"Add State(s) to Queue__jki_lib_state_machine.vi"("State(s) in (\"\")"=w297, "State(s) at Back (\"\")"=w291) -> ("States Out"=w296:string)  [unwired: 13 in]
            n106 = call <vilib>:"Add State(s) to Queue__jki_lib_state_machine.vi"("State(s) in Front (\"\")"=w296, "State(s) in (\"\")"=w302) -> ("States Out"=w301:string)  [unwired: 13 in]
          }
          frame "Macro: Post Error Handling" {
            # "Clear Last Error?"
            n107 = Unbundle By Name(w309) -> ("Core.Last Error.remaining states"=w311:string, "Core.Shutdown?"=w312:bool)
            n108 = Unbundle By Name(w309) -> ("Core.Last Error.error"=w304:errorcluster)
            n109 = case shown="False" FALSE {
              tunnel: w304 -> [w315 _]
              tunnel: [w315 _] -> w303
              frame False {
              }
              frame True {
              }
            }
            n110 = case shown="True" w312 {
              tunnel: w311 -> [w316 w318]
              tunnel: [w316 w317] -> w308
              frame False {
                # "These are the remaining states (at the moment the error occured). States can be altered according to business logic."
                # "NOT SHUTTING DOWN"
              }
              frame True {
                # "Developer can decide to alter the states but should be aware that during the shutdown process, there are certain states that must be run for the SMO to properly shut itself (and this process) down. As such, one can add states to perform additional clean-ups, but should append the remaining state to be executed."
                # "SHUTTING DOWN"
                n111 = call <vilib>:"Add State(s) to Queue__jki_lib_state_machine.vi"("State(s) in (\"\")"=w318) -> ("States Out"=w317:string)  [unwired: 14 in]
              }
            }
            n112 = Bundle By Name(cluster=w309, "Core.Last Error.error"=w303) -> (w310:T7)
            n113 = call <vilib>:"Add State(s) to Queue__jki_lib_state_machine.vi"("State(s) in Front (\"\")"=w308, "State(s) in (\"\")"=w306) -> ("States Out"=w307:string)  [unwired: 13 in]
          }
          frame "---------- Process ----------" {
            # "Template Separator\n(You can make a copy of, or modify, this frame)"
            n114 = call <vilib>:"Add State(s) to Queue__jki_lib_state_machine.vi"("State(s) in (\"\")"=w323) -> ("States Out"=w322:string)  [unwired: 14 in]
          }
          frame "Process: Sync" {
            n115 = Unbundle By Name(w331) -> ("SelfRef"=w327:refnum<class "Instrument.lvclass">)
            n116 = call <vilib>:"WaitOnProcessSync.vi"("error in (no error)"=w326, "SMO"=w327) -> ("error out"=w325:errorcluster, "Don't run?"=w330:bool)  [unwired: 7 in, 1 out]
            n117 = Select(t="Data: Cleanup\nEvents: Unregister\nExit", s=w330, f="") -> (s? t:f=w324:string)
            n118 = call <vilib>:"Add State(s) to Queue__jki_lib_state_machine.vi"("State(s) in Front (\"\")"=w324, "State(s) in (\"\")"=w334) -> ("States Out"=w333:string)  [unwired: 13 in]
          }
          frame "Process: SelfTerminate" {
            # "Template Separator\n(You can make a copy of, or modify, this frame)"
            n119 = Unbundle By Name(w338) -> ("SelfRef"=w340:refnum<class "Instrument.lvclass">)
            n120 = call <vilib>:"SelfTerminate.vi"("error in (no error)"=w336, "SMO in"=w340) -> ("error out"=w335:errorcluster, "SMO out"=w339:refnum<class "Instrument.lvclass">)  [unwired: 8 in]
            n121 = Bundle By Name(cluster=w338, "SelfRef"=w339) -> (w337:T7)
            n122 = call <vilib>:"Add State(s) to Queue__jki_lib_state_machine.vi"("State(s) in (\"\")"=w343) -> ("States Out"=w342:string)  [unwired: 14 in]
          }
          frame "---------- Events ----------" {
            # "Template Separator\n(You can make a copy of, or modify, this frame)"
            n123 = call <vilib>:"Add State(s) to Queue__jki_lib_state_machine.vi"("State(s) in (\"\")"=w348) -> ("States Out"=w347:string)  [unwired: 14 in]
          }
          frame "Events: Register" {
            n124 = Unbundle By Name(w377) -> ("SelfRef"=w372:refnum<class "Instrument.lvclass">, "Dependencies.RemoteControl"=w371:refnum<class "RemoteControl.lvclass">, "Dependencies.Logger.PGSQL"=w366:refnum<class "Logger.PGSQL.lvclass">, "Dependencies.Logger.Error"=w367:refnum<class "Logger.Error.lvclass">)
            n125 = call <vilib>:"GetProtectedEvents.vi"("SMO"=w372) -> ("error out"=w374:errorcluster, "SMO Protected Events"=w362:T10, "SMO out"=w365:refnum<class "Instrument.lvclass">)  [unwired: 8 in]
            n126 = call "Instrument.GetPrivateEvents.vi"("Instrument"=w365) -> ("error out"=w361:errorcluster, "Instrument Private Events"=w359:T11)  [unwired: 8 in, 1 out]
            n127 = call <userlib>:"RemoteControl.GetPublicEvents.vi"("RemoteControl"=w371) -> ("error out"=w360:errorcluster, "RC Public Events"=w358:T12, "RemoteControl out"=w364:refnum<class "RemoteControl.lvclass">)  [unwired: 8 in]
            n128 = call <vilib>:"GetPublicEvents.vi"("SMO"=w364) -> ("error out"=w370:errorcluster, "Public Events"=w357:T13)  [unwired: 8 in, 1 out]
            n129 = call <vilib>:"GetPublicEvents.vi"("SMO"=w366) -> ("error out"=w369:errorcluster, "Public Events"=w355:T13)  [unwired: 8 in, 1 out]
            n130 = call <vilib>:"GetPublicEvents.vi"("SMO"=w367) -> ("error out"=w368:errorcluster, "Public Events"=w352:T13)  [unwired: 8 in, 1 out]
            n131 = call "Rename RC SMO Private Events.vi"("error in (no error)"=w370, "Public Events"=w357) -> ("error out"=w349:errorcluster, "RC SMO Public Events"=w356:T13)  [unwired: 8 in]
            n132 = call "Rename PGSQL SMO Private Events.vi"("error in (no error)"=w369, "Public Events"=w355) -> ("error out"=w350:errorcluster, "PGSQL SMO Public Events"=w354:T13)  [unwired: 8 in]
            n133 = call "Rename Error SMO Private Events.vi"("error in (no error)"=w368, "Public Events"=w352) -> ("error out"=w353:errorcluster, "Error SMO Public Events"=w351:T13)  [unwired: 8 in]
            n134 = register-events(w362, w359, w358, w356, w354, w351) -> (reference out=w376:refnum<event-registration>, error out=w363:errorcluster)  [unwired: 2 in]
            n135 = Merge Errors(w363, w349, w350, w353, w360, w361, w374, w373) -> (w375:errorcluster)
            n136 = call <vilib>:"Add State(s) to Queue__jki_lib_state_machine.vi"("State(s) in (\"\")"=w379) -> ("States Out"=w378:string)  [unwired: 14 in]
          }
          frame "Events: Unregister" {
            n137 = Unregister For Events(event registration refnum=w382, error in=w381) -> (error out=w380:errorcluster)
            n138 = call <vilib>:"Clear Errors.vi"("error in (no error)"=w380) -> ()  [unwired: 5 in, 2 out]
            n139 = call <vilib>:"Add State(s) to Queue__jki_lib_state_machine.vi"("State(s) in (\"\")"=w385) -> ("States Out"=w384:string)  [unwired: 14 in]
          }
          frame "---------- Instrument ----------" {
            n140 = call <vilib>:"Add State(s) to Queue__jki_lib_state_machine.vi"("State(s) in (\"\")"=w390) -> ("States Out"=w389:string)  [unwired: 14 in]
          }
          frame "Instrument: Handle Remote Command" {
            # "parse and handle incoming commands\n- respond with data on hand\n- forward message to child instrument...etc"
            n141 = Unbundle By Name(w401) -> ("Dependencies.RemoteControl"=w406:refnum<class "RemoteControl.lvclass">, "SelfRef"=w403:refnum<class "Instrument.lvclass">, "Message.Command"=w402:string, "Message.Data"=w398:variant, "Message.ID"=w404:string)
            "Remote Command" <- w402
            n142 = call-dynamic "Handle Command.vi"("error in (no error)"=w405, "Data"=w398, "Command"=w402, "Instrument in"=w403) -> ("error out"=w391:errorcluster, "Processed Data"=w394:variant, "Command"=w393:string, "Instrument out"=w399:refnum<class "Instrument.lvclass">)  [unwired: 4 in]
            n143 = Empty String/Path?(string/path=w393) -> (empty?=w397:bool)
            n144 = Empty String/Path?(string/path=w394) -> (empty?=w396:bool)
            n145 = And(x=w397, y=w396) -> (x .and. y?=w395:bool)
            n146 = case shown="False" w395 {
              tunnel: w406 -> [w417 _]
              tunnel: w391 -> [w413 w418]
              tunnel: w394 -> [w415 _]
              tunnel: w404 -> [w416 _]
              tunnel: [w412 w418] -> w392
              tunnel: w393 -> [w414 _]
              frame False {
                # "command respond"
                n147 = Bundle By Name(cluster=T3 {"Command"="", "Data"=variant(string ""), "ID"=""} ("Message"), "Command"=w414, "Data"=w415, "ID"=w416) -> (w410:T3)
                n148 = call <userlib>:"RemoteControl.SendMessageToProcess.vi"("error in (no error)"=w413, "Message"=w410, "RemoteControl"=w417) -> ("error out"=w412:errorcluster)  [unwired: 7 in, 1 out]
              }
              frame True {
              }
            }
            n149 = Bundle By Name(cluster=w401, "SelfRef"=w399) -> (w400:T7)
            n150 = call <vilib>:"Add State(s) to Queue__jki_lib_state_machine.vi"("State(s) in (\"\")"=w409) -> ("States Out"=w408:string)  [unwired: 14 in]
          }
          frame "Instrument: Handle Local Command" {
            # "parse and handle incoming commands\n- respond with data on hand\n- forward message to child instrument...etc"
            n151 = Unbundle By Name(w426) -> ("SelfRef"=w432:refnum<class "Instrument.lvclass">, "Message.Command"=w428:string, "Message.Data"=w433:variant, "Message.ID"=w427:string)
            "Local Command" <- w428
            n152 = call-dynamic "Handle Command.vi"("error in (no error)"=w434, "Data"=w433, "Command"=w428, "Instrument in"=w432) -> ("error out"=w430:errorcluster, "Processed Data"=w419:variant, "Command"=w420:string, "Instrument out"=w429:refnum<class "Instrument.lvclass">)  [unwired: 4 in]
            n153 = Empty String/Path?(string/path=w420) -> (empty?=w423:bool)
            n154 = Empty String/Path?(string/path=w419) -> (empty?=w422:bool)
            n155 = And(x=w423, y=w422) -> (x .and. y?=w421:bool)
            n156 = case shown="False" w421 {
              tunnel: [w439 w440] -> w431
              tunnel: w430 -> [w439 w441]
              tunnel: w429 -> [w438 w446]
              tunnel: w419 -> [_ w445]
              tunnel: w427 -> [_ w444]
              tunnel: [w438 w443] -> w424
              tunnel: w420 -> [_ w442]
              frame True {
              }
              frame False {
                # "command response"
                n157 = call "Instrument.MessageFromProcess.vi"("ID"=w444, "error in (no error)"=w441, "Data"=w445, "Command"=w442, "Instrument"=w446) -> ("error out"=w440:errorcluster, "Instrument out"=w443:refnum<class "Instrument.lvclass">)  [unwired: 5 in]
              }
            }
            n158 = Bundle By Name(cluster=w426, "SelfRef"=w424) -> (w425:T7)
            n159 = call <vilib>:"Add State(s) to Queue__jki_lib_state_machine.vi"("State(s) in (\"\")"=w437) -> ("States Out"=w436:string)  [unwired: 14 in]
          }
          frame "Instrument: getAll" {
            # "do this and can change dynamically\n(after running Inst Open for example)"
            # "get all parameters from the instrument"
            n160 = Unbundle By Name(w451) -> ("SelfRef"=w457:refnum<class "Instrument.lvclass">)
            n161 = call-dynamic "Handle Command.vi"("error in (no error)"=w458, "Command"="getAll", "Instrument in"=w457) -> ("error out"=w456:errorcluster, "Processed Data"=w449:variant, "Command"=w453:string, "Instrument out"=w452:refnum<class "Instrument.lvclass">)  [unwired: 5 in]
            n162 = case shown="Default" w453 {
              selector: w453 -> [w469 _]
              tunnel: w449 -> [w464 _]
              tunnel: w456 -> [w468 w473]
              tunnel: [w465 w473] -> w455
              tunnel: w452 -> [w470 w471]
              tunnel: [w463 "" ("Paths")] -> w448
              tunnel: [w462 w471] -> w447
              frame Default {
                # "broadcast update to\nsubscribers (UI. Could be logger)"
                # "call data logger SMO"
                n163 = call "Instrument.MessageFromProcess.vi"("error in (no error)"=w468, "Data"=w464, "Command"=w469, "Instrument"=w470) -> ("error out"=w466:errorcluster, "Instrument out"=w467:refnum<class "Instrument.lvclass">)  [unwired: 6 in]
                n164 = call-dynamic "Get SMO PGSQL Log Paths.vi"("error in (no error)"=w466, "Instrument in"=w467) -> ("error out"=w465:errorcluster, "Paths"=w463:string, "Instrument out"=w462:refnum<class "Instrument.lvclass">)  [unwired: 7 in]
              }
              frame "" {
                # "do nothing if command is empty"
              }
            }
            n165 = Bundle By Name(cluster=w451, "getAll"=w449, "Message.Data"=w449, "SelfRef"=w447, "PGSQL.Address"=w448) -> (w450:T7)
            n166 = call <vilib>:"Add State(s) to Queue__jki_lib_state_machine.vi"("State(s) in (\"\")"=w461) -> ("States Out"=w460:string)  [unwired: 14 in]
          }
          frame "Instrument: Log to PGSQL" {
            # "send event to PGSQL process"
            n167 = Unbundle By Name(w476) -> ("Dependencies.Logger.PGSQL"=w479:refnum<class "Logger.PGSQL.lvclass">, "PGSQL.Address"=w475:string, "Message.Data"=w474:variant)
            n168 = call "Logger.PGSQL.WriteVariable.vi"("error in (no error)"=w478, "Data"=w474, "Address"=w475, "Logger"=w479) -> ("error out"=w477:errorcluster)  [unwired: 6 in, 1 out]
            n169 = call <vilib>:"Add State(s) to Queue__jki_lib_state_machine.vi"("State(s) in (\"\")"=w482) -> ("States Out"=w481:string)  [unwired: 14 in]
          }
          frame "Instrument: Open" {
            n170 = Unbundle By Name(w487) -> ("SelfRef"=w486:refnum<class "Instrument.lvclass">)
            n171 = disable-structure shown="Enabled" {
              disable-tunnel: w486 -> [w495 w497]
              disable-tunnel: [w494 w497] -> w485
              disable-tunnel: [w493 w496] -> w484
              disable-tunnel: w483 -> [w492 w496]
              frame Disabled {
                # "This case is enabled by default in Instrument Framework pre-v1.13.\nIf you have not yet updated your code (open/close should go into the child process.vi) then enable this case"
                n172 = call-dynamic "Open Hardware.vi"("error in (no error)"=w492, "Instrument in"=w495) -> ("error out"=w493:errorcluster, "Instrument out"=w494:refnum<class "Instrument.lvclass">)  [unwired: 8 in]
              }
              frame Enabled {
              }
            }
            n173 = Bundle By Name(cluster=w487, "SelfRef"=w485) -> (w488:T7)
            n174 = call <vilib>:"Add State(s) to Queue__jki_lib_state_machine.vi"("State(s) in (\"\")"=w491) -> ("States Out"=w490:string)  [unwired: 14 in]
          }
          frame "Instrument: Close" {
            n175 = Unbundle By Name(w500) -> ("SelfRef"=w503:refnum<class "Instrument.lvclass">)
            n176 = disable-structure shown="Disabled" {
              disable-tunnel: w503 -> [w510 w512]
              disable-tunnel: [w509 w512] -> w502
              disable-tunnel: [w508 w511] -> w499
              disable-tunnel: w498 -> [w507 w511]
              frame Disabled {
                # "This case is enabled by default in Instrument Framework pre-v1.13.\nIf you have not yet updated your code (open/close should go into the child process.vi) then enable this case"
                n177 = call-dynamic "Close Hardware.vi"("error in (no error)"=w507, "Instrument in"=w510) -> ("error out"=w508:errorcluster, "Instrument out"=w509:refnum<class "Instrument.lvclass">)  [unwired: 8 in]
              }
              frame Enabled {
              }
            }
            n178 = Bundle By Name(cluster=w500, "SelfRef"=w502) -> (w501:T7)
            n179 = call <vilib>:"Add State(s) to Queue__jki_lib_state_machine.vi"("State(s) in (\"\")"=w506) -> ("States Out"=w505:string)  [unwired: 14 in]
          }
        }
      }
    }
    frame Error {
    }
  }
  n180 = call-parent "Process.vi"("error in"=w5, "SMO"=w4) -> ("error out"=w2:errorcluster, "SMO out"=→"Instrument out":refnum<class "Instrument.lvclass">)  [unwired: 8 in]
  n181 = Merge Errors(w2, w1) -> (→"error out":errorcluster)
